vi "oldbis בדיקת מפל מתח בין הדקי הממסר תחת עומס 5.vi"(8 "error":errorcluster, 10 "lines":tag="PXI1Slot8/port0/line1", 11 "Path for Log":path) -> (0 "error IO":errorcluster, 1 "In Range?":bool, 2 "מפל מתח בין דקי הממסר תחת עומס":dbl, 3 "תוצאה זמנית":dbl)   [LabVIEW 2014]
uses:
  M9700 Driver/85/vi.lib/M9700 Modbus.llb/CTL Register Address.ctl
  M9700 Driver/86/vi.lib/M9700 Modbus.llb/CTL CMD Register.ctl
  <vilib>/Instr/_visa.llb/VISA Configure Serial Port (Instr).vi
  <vilib>/DAQmx/create/channels.llb/DAQmx Create Channel (DO-Digital Output).vi
  <vilib>/DAQmx/write.llb/DAQmx Write (Digital Bool 1Line 1Point).vi
panel:
  out "progress":dbl(slide) min=0.0 max=10.0 scale=0.0..10.0
  in  "stop":bool
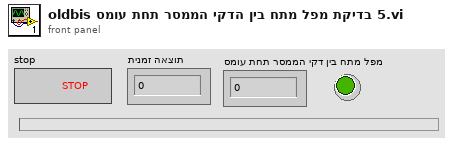
[diagram p1: front panel]
types:
  T1 = enum32{"Invalid", "Standard", "Closed", "Hidden", "Minimized", "Maximized"}
  T2 = typedef "CTL CMD Register.ctl" = u8
  T3 = typedef "CTL Register Address.ctl" = u16
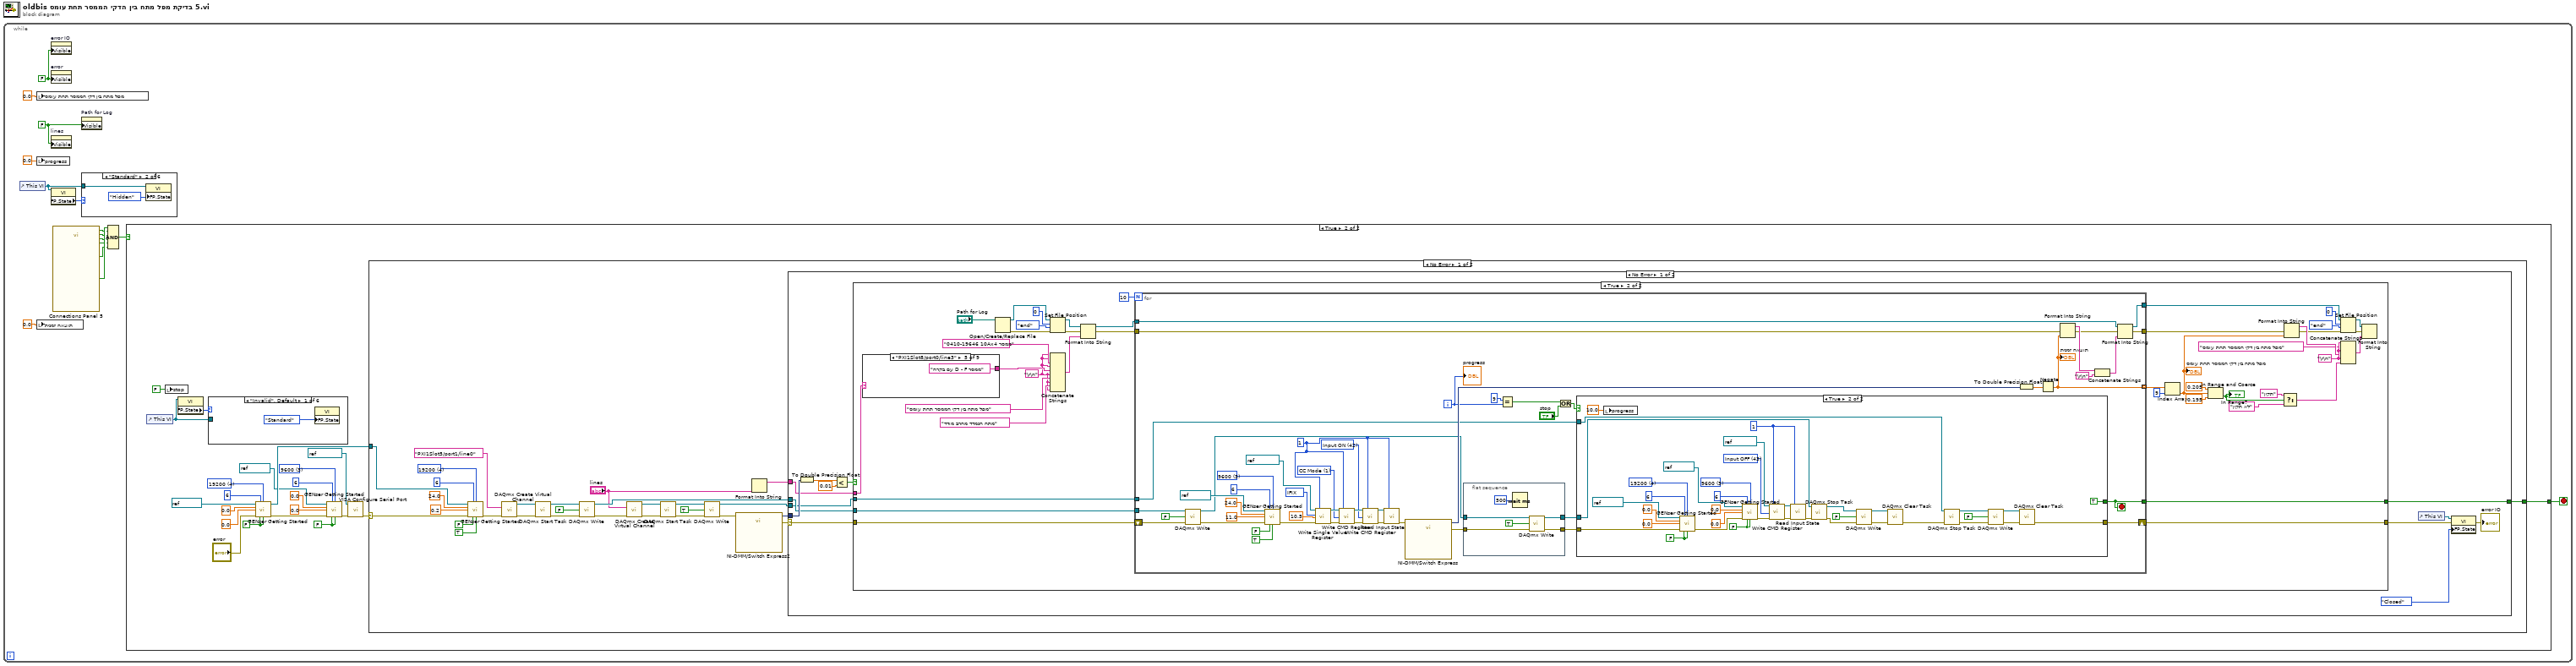
[diagram p0: block diagram]
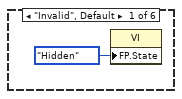
[diagram p2: hidden frame]
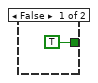
[diagram p7: hidden frame]
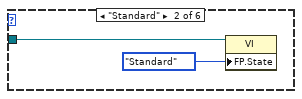
[diagram p8: hidden frame]
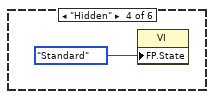
[diagram p10: hidden frame]
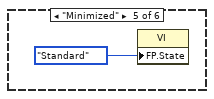
[diagram p11: hidden frame]
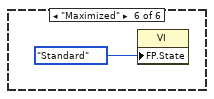
[diagram p12: hidden frame]
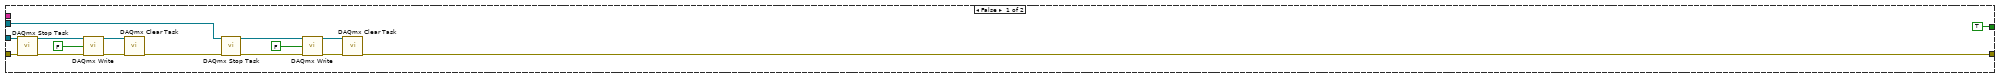
[diagram p13: hidden frame]
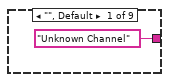
[diagram p14: hidden frame]
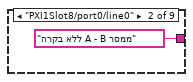
[diagram p15: hidden frame]
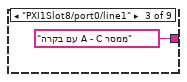
[diagram p16: hidden frame]
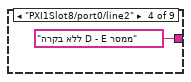
[diagram p17: hidden frame]
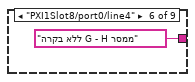
[diagram p18: hidden frame]
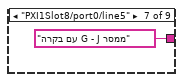
[diagram p19: hidden frame]
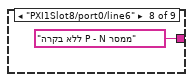
[diagram p20: hidden frame]
diagram:
  n1 = while {
    stop <- w15 stop-if-true
    w3 = FALSE ("Visible")
    w10 = FALSE ("Visible")
    n2 = control-ref of="This VI"() -> (w2:refnum<vi>)
    n3 = local write "מפל מתח בין דקי הממסר תחת עומס"(0.0 ("מפל מתח בין דקי הממסר תחת עומס")) -> ()
    n4 = local write "progress"(0.0 ("progress")) -> ()
    n5 = local write "תוצאה זמנית"(0.0 ("תוצאה זמנית")) -> ()
    n6 = property on="error IO" class="Clust (strict)"("Visible"=w10) -> ()  [unwired: 2 in, 2 out]
    n7 = property on="error" class="Clust (strict)"("Visible"=w10) -> ()  [unwired: 2 in, 2 out]
    n8 = property on="lines" class="DAQmxName"("Visible"=w3) -> ()  [unwired: 2 in, 2 out]
    n9 = property class="VI"(reference=w2) -> ("FP.State"=w1:T1)  [unwired: 1 in, 2 out]
    n10 = call "Connections Panel 5.vi"() -> ("Input Name 10"=w4:bool, "Input Name 6"=w8:bool, "Input Name 7"=w7:bool, "Input Name 8"=w6:bool, "Input Name 9"=w5:bool, "OK"=w9:bool)  [unwired: 13 in, 1 out]
    n11 = property on="Path for Log" class="Path"("Visible"=w3) -> ()  [unwired: 2 in, 2 out]
    n12 = case shown="\"Standard\"" w1 {
      tunnel: w2 -> [_ w17 _ _ _ _]
      frame "Invalid", Default {
        n13 = property class="VI"("FP.State"=T1."Hidden" ("Front Panel Window:State")) -> ()  [unwired: 2 in, 2 out]
      }
      frame "Standard" {
        n14 = property class="VI"(reference=w17, "FP.State"=T1."Hidden" ("Front Panel Window:State")) -> ()  [unwired: 1 in, 2 out]
      }
      frame "Closed" {
      }
      frame "Hidden" {
      }
      frame "Minimized" {
      }
      frame "Maximized" {
      }
    }
    n15 = Compound Arithmetic op=AND(w9, w8, w7, w6, w5, w4) -> (w14:bool)
    n16 = case shown="True" w14 {
      tunnel: [TRUE w28] -> w15
      frame False {
      }
      frame True {
        w24 = FALSE ("Reset (T)")
        w33 = u16 3 items=["1200", "2400", "4800", "9600", "19200"] ("BAUD")
        w23 = FALSE ("Output On (T)")
        w38 = u16 4 items=["1200", "2400", "4800", "9600", "19200"] ("BAUD")
        n17 = control-ref of="This VI"() -> (w20:refnum<vi>)
        n18 = local write "stop"(FALSE ("stop")) -> ()
        n19 = property class="VI"(reference=w20) -> ("FP.State"=w21:T1)  [unwired: 1 in, 2 out]
        n20 = case shown="\"Invalid\", Default" w21 {
          tunnel: w20 -> [_ w43 _ _ _ _]
          frame "Invalid", Default {
            n21 = property class="VI"("FP.State"=T1."Standard" ("Front Panel Window:State")) -> ()  [unwired: 2 in, 2 out]
          }
          frame "Standard" {
            n22 = property class="VI"(reference=w43, "FP.State"=T1."Standard" ("Front Panel Window:State")) -> ()  [unwired: 1 in, 2 out]
          }
          frame "Closed" {
          }
          frame "Hidden" {
            n23 = property class="VI"("FP.State"=T1."Standard" ("Front Panel Window:State")) -> ()  [unwired: 2 in, 2 out]
          }
          frame "Minimized" {
            n24 = property class="VI"("FP.State"=T1."Standard" ("Front Panel Window:State")) -> ()  [unwired: 2 in, 2 out]
          }
          frame "Maximized" {
            n25 = property class="VI"("FP.State"=T1."Standard" ("Front Panel Window:State")) -> ()  [unwired: 2 in, 2 out]
          }
        }
        n26 = call "GENser Getting Started.vi"("VISA"=refnum<visa-resource-name> "COM6", "GEN Addr"=i16 6, "BAUD"=w38, "Voltage Limit"=0.0, "Current Limit"=0.0, "error"="error", "Reset (T)"=w23, "Output On (T)"=w23) -> ("VISA out"=w40:refnum<visa-resource-name>, "error out"=w29:errorcluster)  [unwired: 4 in, 2 out]
        n27 = call "GENser Getting Started.vi"("VISA"=refnum<visa-resource-name> "COM4", "GEN Addr"=i16 6, "BAUD"=w33, "Voltage Limit"=0.0, "Current Limit"=0.0, "error"=w29, "Reset (T)"=w24, "Output On (T)"=w24) -> ("error out"=w26:errorcluster)  [unwired: 4 in, 3 out]
        n28 = call-poly "VISA Configure Serial Port"("VISA resource name"=refnum<visa-resource-name> "COM13", "error in (no error)"=w26) -> ("error out"=w25:errorcluster)  [unwired: 4 in, 9 out]
        n29 = case shown="No Error" w25 {
          selector: w25 -> [w73 _]
          tunnel: w40 -> [w76 _]
          tunnel: [w75 w255] -> w28
          frame No Error {
            w67 = u16 4 items=["1200", "2400", "4800", "9600", "19200"] ("BAUD")
            n30 = call "GENser Getting Started.vi"("VISA"=w76, "GEN Addr"=i16 6, "BAUD"=w67, "Voltage Limit"=24.0, "Current Limit"=0.2, "error"=w73, "Reset (T)"=FALSE, "Output On (T)"=TRUE) -> ("error out"=w61:errorcluster)  [unwired: 4 in, 3 out]
            n31 = call-poly <vilib>:"DAQmx Create Virtual Channel.vi"("lines"=tag "PXI1Slot5/port1/line0", "error in"=w61) -> ("task out"=w57:refnum<k21>, "error out"=w58:errorcluster)  [unwired: 12 in]
            n32 = call <vilib>:"DAQmx Start Task.vi"("task/channels in"=w57, "error in"=w58) -> ("task out"=w55:refnum<k21>, "error out"=w54:errorcluster)  [unwired: 12 in]
            n33 = call-poly <vilib>:"DAQmx Write.vi"("task/channels in"=w55, "data"=FALSE, "error in"=w54) -> ("task out"=w65:refnum<k21>, "error out"=w64:errorcluster)  [unwired: 10 in, 1 out]
            n34 = call-poly <vilib>:"DAQmx Create Virtual Channel.vi"("lines"="lines", "error in"=w64) -> ("task out"=w48:refnum<k21>, "error out"=w49:errorcluster)  [unwired: 12 in]
            n35 = call <vilib>:"DAQmx Start Task.vi"("task/channels in"=w48, "error in"=w49) -> ("task out"=w51:refnum<k21>, "error out"=w50:errorcluster)  [unwired: 12 in]
            n36 = call-poly <vilib>:"DAQmx Write.vi"("task/channels in"=w51, "data"=TRUE, "error in"=w50) -> ("task out"=w63:refnum<k21>, "error out"=w60:errorcluster)  [unwired: 10 in, 1 out]
            n37 = call "NI-DMM/Switch Express2"("error in"=w60) -> ("signals out"=w74:dynamicdata, "error out"=w59:errorcluster)  [unwired: 16 in, 1 out]
            n38 = Format Into String("lines") -> (resulting string=w66:string)  [unwired: 3 in, 1 out]
            n39 = case shown="No Error" w59 {
              selector: w59 -> [w87 _]
              tunnel: [w86 w250] -> w75
              tunnel: w74 -> [w89 _]
              tunnel: w65 -> [w80 _]
              tunnel: w66 -> [w78 _]
              tunnel: w63 -> [w77 _]
              frame No Error {
                n40 = To Double Precision Float(number=w89) -> (double precision float=w85:dbl)
                n41 = Less?(x=w85, y=0.01) -> (x < y?=w88:bool)
                n42 = case shown="True" w88 {
                  tunnel: w87 -> [w93 w108]
                  tunnel: [TRUE w146] -> w86
                  tunnel: [w90 w140] -> w81
                  tunnel: w80 -> [w92 w141]
                  tunnel: w78 -> [_ w110]
                  tunnel: w77 -> [w91 w109]
                  frame False {
                    n43 = call <vilib>:"DAQmx Stop Task.vi"("task/channels in"=w92, "error in"=w93) -> ("task out"=w104:refnum<k21>, "error out"=w102:errorcluster)  [unwired: 12 in]
                    n44 = call-poly <vilib>:"DAQmx Write.vi"("task/channels in"=w104, "data"=FALSE, "error in"=w102) -> ("task out"=w101:refnum<k21>, "error out"=w100:errorcluster)  [unwired: 10 in, 1 out]
                    n45 = call <vilib>:"DAQmx Clear Task.vi"("task in"=w101, "error in"=w100) -> ("error out"=w94:errorcluster)  [unwired: 13 in]
                    n46 = call <vilib>:"DAQmx Stop Task.vi"("task/channels in"=w91, "error in"=w94) -> ("task out"=w99:refnum<k21>, "error out"=w97:errorcluster)  [unwired: 12 in]
                    n47 = call-poly <vilib>:"DAQmx Write.vi"("task/channels in"=w99, "data"=FALSE, "error in"=w97) -> ("task out"=w96:refnum<k21>, "error out"=w95:errorcluster)  [unwired: 10 in, 1 out]
                    n48 = call <vilib>:"DAQmx Clear Task.vi"("task in"=w96, "error in"=w95) -> ("error out"=w90:errorcluster)  [unwired: 13 in]
                  }
                  frame True {
                    w127 = "\r\n"
                    w106 = "\r\n"
                    n49 = case shown="\"PXI1Slot8/port0/line3\"" w110 {
                      tunnel: ["Unknown Channel" "ללא בקרה A - B ממסר" "עם בקרה A - C ממסר" "ללא בקרה D - E ממסר" "עם בקרה D - F ממסר" "ללא בקרה G - H ממסר" "עם בקרה G - J ממסר" "ללא בקרה P - N ממסר" "עם בקרה P - L ממסר"] -> w107
                      frame "", Default {
                      }
                      frame "PXI1Slot8/port0/line0" {
                      }
                      frame "PXI1Slot8/port0/line1" {
                      }
                      frame "PXI1Slot8/port0/line2" {
                      }
                      frame "PXI1Slot8/port0/line3" {
                      }
                      frame "PXI1Slot8/port0/line4" {
                      }
                      frame "PXI1Slot8/port0/line5" {
                      }
                      frame "PXI1Slot8/port0/line6" {
                      }
                      frame "PXI1Slot8/port0/line7" {
                      }
                    }
                    n50 = Open/Create/Replace File(file path (use dialog)="Path for Log") -> (refnum out=w137:refnum<file>, error out=w136:errorcluster)  [unwired: 5 in, 1 out]
                    n51 = Set File Position(offset (in bytes) (0)=i64 0, refnum=w137, from (0:start)=enum16{"start", "end", "current"}."end", error in=w136) -> (refnum out=w133:refnum<file>, error out=w130:errorcluster)
                    n52 = Concatenate Strings(w106, w106, "0410-19646 10Ax4 ממסר", w106, w107, w106, "מפל מתח בין דקי הממסר תחת עומס", w106, "מתח הנמדד מהרב מודד", w106) -> (w135:string)
                    n53 = Format Into String(initial string=w133, error in=w130, w135) -> (resulting string=w128:refnum<file>, error out=w129:errorcluster)  [unwired: 1 in]
                    n54 = for {
                      N: 10 -> [_]
                      tunnel: [w180] -> w146
                      shift-right: [w177] -> w140
                      shift-left: w108 -> [w172]
                      tunnel: [w158] -> w145 mode=indexing
                      tunnel: w141 -> [w173]
                      tunnel: w129 -> [w162]
                      tunnel: w128 -> [w164]
                      tunnel: [w161] -> w121
                      tunnel: [w160] -> w112
                      tunnel: w109 -> [w159]
                      i -> [w176]
                      stop <- w180 stop-if-true
                      w188 = T2 42 items=["CC Mode"=1, "CV Mode"=2, "CW Mode"=3, "CR Mode"=4, "Short Mode"=26, "Set SysPara"=41, "Input ON"=42, "Input OFF"=43] ("CMD Register Value")
                      w191 = u8 1 ("Load Address")
                      w195 = T2 1 items=["CC Mode"=1, "CV Mode"=2, "CW Mode"=3, "CR Mode"=4, "Short Mode"=26, "Set SysPara"=41, "Input ON"=42, "Input OFF"=43] ("CMD Register Value")
                      w198 = T3 2561 items=["REMOTE"=1283, "ISTATE"=1296, "CMD"=2560, "IFIX"=2561, "UFIX"=2563, "PFIX"=2565, "RFIX"=2567, "IMAX"=2612, "UMAX"=2614, "PMAX"=2616, "U"=2816, "I"=2818, "MODEL"=2822, "EDITION"=2823] ("Register Address")
                      w203 = u16 3 items=["1200", "2400", "4800", "9600", "19200"] ("BAUD")
                      n55 = call-poly <vilib>:"DAQmx Write.vi"("task/channels in"=w173, "data"=FALSE, "error in"=w172) -> ("task out"=w171:refnum<k21>, "error out"=w170:errorcluster)  [unwired: 10 in, 1 out]
                      n56 = call "GENser Getting Started.vi"("VISA"=refnum<visa-resource-name> "COM4", "GEN Addr"=i16 6, "BAUD"=w203, "Voltage Limit"=24.0, "Current Limit"=11.0, "error"=w170, "Reset (T)"=FALSE, "Output On (T)"=TRUE) -> ("error out"=w193:errorcluster)  [unwired: 4 in, 3 out]
                      n57 = call "Write Single Value Register.vi"("VISA resource name"=refnum<visa-resource-name> "COM13", "Starting Address(HEX)"=w198, "Register Single Value"=sgl 10.5, "error in"=w193, "Load Address"=w191) -> ("VISA resource name out"=w197:refnum<visa-resource-name>, "error out"=w196:errorcluster)  [unwired: 13 out]
                      n58 = call "Write CMD Register.vi"("VISA resource name"=w197, "CMD Value"=w195, "error in"=w196, "Load Address"=w191) -> ("VISA resource name out"=w192:refnum<visa-resource-name>, "error out"=w189:errorcluster)  [unwired: 14 out]
                      n59 = call "Write CMD Register.vi"("VISA resource name"=w192, "CMD Value"=w188, "error in"=w189, "Load Address"=w191) -> ("VISA resource name out"=w190:refnum<visa-resource-name>, "error out"=w187:errorcluster)  [unwired: 14 out]
                      n60 = call "Read Input State.vi"("VISA resource name"=w190, "error in"=w187, "Load Address"=w191) -> ("error out"=w186:errorcluster)  [unwired: 16 out]
                      n61 = call "NI-DMM/Switch Express"("error in"=w186) -> ("signals out"=w185:dynamicdata, "error out"=w174:errorcluster)  [unwired: 16 in, 1 out]
                      n62 = flat-sequence {
                        tunnel: [w210] -> w175
                        tunnel: w174 -> [w209]
                        tunnel: w171 -> [w207]
                        tunnel: [w206] -> w168
                        frame #0 {
                          n63 = Wait (ms)(milliseconds to wait=u32 500) -> ()  [unwired: 1 out]
                          n64 = call-poly <vilib>:"DAQmx Write.vi"("task/channels in"=w207, "data"=TRUE, "error in"=w209) -> ("task out"=w206:refnum<k21>, "error out"=w210:errorcluster)  [unwired: 10 in, 1 out]
                        }
                      }
                      n65 = Equal?(x=9, y=w176) -> (x = y?=w182:bool)
                      n66 = Or(x=w182, y="stop") -> (x .or. y?=w183:bool)
                      n67 = case shown="True" w183 {
                        tunnel: [FALSE TRUE] -> w180
                        tunnel: w175 -> [w211 w238]
                        tunnel: [w211 w215] -> w177
                        tunnel: w168 -> [_ w221]
                        tunnel: w159 -> [_ w213]
                        frame False {
                        }
                        frame True {
                          w229 = u8 1 ("Load Address")
                          w232 = T2 43 items=["CC Mode"=1, "CV Mode"=2, "CW Mode"=3, "CR Mode"=4, "Short Mode"=26, "Set SysPara"=41, "Input ON"=42, "Input OFF"=43] ("CMD Register Value")
                          w236 = FALSE ("Reset (T)")
                          w242 = u16 3 items=["1200", "2400", "4800", "9600", "19200"] ("BAUD")
                          w235 = FALSE ("Reset (T)")
                          w245 = u16 4 items=["1200", "2400", "4800", "9600", "19200"] ("BAUD")
                          n68 = local write "progress"(10.0 ("progress")) -> ()
                          n69 = call "GENser Getting Started.vi"("VISA"=refnum<visa-resource-name> "COM6", "GEN Addr"=i16 6, "BAUD"=w245, "Voltage Limit"=0.0, "Current Limit"=0.0, "error"=w238, "Reset (T)"=w235, "Output On (T)"=w235) -> ("error out"=w237:errorcluster)  [unwired: 4 in, 3 out]
                          n70 = call "GENser Getting Started.vi"("VISA"=refnum<visa-resource-name> "COM4", "GEN Addr"=i16 6, "BAUD"=w242, "Voltage Limit"=0.0, "Current Limit"=0.0, "error"=w237, "Reset (T)"=w236, "Output On (T)"=w236) -> ("error out"=w234:errorcluster)  [unwired: 4 in, 3 out]
                          n71 = call "Write CMD Register.vi"("VISA resource name"=refnum<visa-resource-name> "COM13", "CMD Value"=w232, "error in"=w234, "Load Address"=w229) -> ("VISA resource name out"=w230:refnum<visa-resource-name>, "error out"=w233:errorcluster)  [unwired: 14 out]
                          n72 = call "Read Input State.vi"("VISA resource name"=w230, "error in"=w233, "Load Address"=w229) -> ("error out"=w222:errorcluster)  [unwired: 16 out]
                          n73 = call <vilib>:"DAQmx Stop Task.vi"("task/channels in"=w221, "error in"=w222) -> ("task out"=w227:refnum<k21>, "error out"=w225:errorcluster)  [unwired: 12 in]
                          n74 = call-poly <vilib>:"DAQmx Write.vi"("task/channels in"=w227, "data"=FALSE, "error in"=w225) -> ("task out"=w224:refnum<k21>, "error out"=w223:errorcluster)  [unwired: 10 in, 1 out]
                          n75 = call <vilib>:"DAQmx Clear Task.vi"("task in"=w224, "error in"=w223) -> ("error out"=w214:errorcluster)  [unwired: 13 in]
                          n76 = call <vilib>:"DAQmx Stop Task.vi"("task/channels in"=w213, "error in"=w214) -> ("task out"=w220:refnum<k21>, "error out"=w218:errorcluster)  [unwired: 12 in]
                          n77 = call-poly <vilib>:"DAQmx Write.vi"("task/channels in"=w220, "data"=FALSE, "error in"=w218) -> ("task out"=w217:refnum<k21>, "error out"=w216:errorcluster)  [unwired: 10 in, 1 out]
                          n78 = call <vilib>:"DAQmx Clear Task.vi"("task in"=w217, "error in"=w216) -> ("error out"=w215:errorcluster)  [unwired: 13 in]
                        }
                      }
                      n79 = To Double Precision Float(number=w185) -> (double precision float=w157:dbl)
                      n80 = Negate(x=w157) -> (-x=w158:dbl)
                      "תוצאה זמנית" <- w158
                      n81 = Format Into String(error in=w162, w158) -> (resulting string=w166:string, error out=w163:errorcluster)  [unwired: 2 in]
                      n82 = Concatenate Strings(w166, "\r\n") -> (w165:string)
                      n83 = Format Into String(initial string=w164, error in=w163, w165) -> (resulting string=w161:refnum<file>, error out=w160:errorcluster)  [unwired: 1 in]
                      "progress" <- w176
                    }
                    n84 = Index Array(array=w145, index=9) -> (element=w120:dbl)
                    "מפל מתח בין דקי הממסר תחת עומס" <- w120
                    n85 = In Range and Coerce(upper limit=0.205, x=w120, lower limit=0.195) -> (In Range?=w115:bool)  [unwired: 1 out]
                    "In Range?" <- w115
                    n86 = Select(t="תקין", s=w115, f="לא תקין") -> (s? t:f=w114:string)
                    n87 = Format Into String(error in=w112, w120) -> (resulting string=w119:string, error out=w113:errorcluster)  [unwired: 2 in]
                    n88 = Set File Position(offset (in bytes) (0)=i64 0, refnum=w121, from (0:start)=enum16{"start", "end", "current"}."end", error in=w113) -> (refnum out=w124:refnum<file>, error out=w123:errorcluster)
                    n89 = Concatenate Strings(w127, "מפל מתח בין דקי הממסר תחת עומס" ("string"), w127, w119, w127, w114) -> (w122:string)
                    n90 = Format Into String(initial string=w124, error in=w123, w122) -> ()  [unwired: 1 in, 2 out]
                  }
                }
                n91 = control-ref of="This VI"() -> (w83:refnum<vi>)
                n92 = property class="VI"(reference=w83, error in=w81, "FP.State"=T1."Closed" ("Front Panel Window:State")) -> (error out=→"error IO":errorcluster)  [unwired: 1 out]
              }
              frame Error {
                n93 = Two Button Dialog(message="בעיית דגימת נתונים ע\"י הכרטיס רב מודד", 1:"ביטול" ("F button name (\"Cancel\")"), 2:"נסה שוב" ("T button name (\"OK\")")) -> (T button?=w251:bool)
                n94 = Not(x=w251) -> (.not. x?=w250:bool)
              }
            }
          }
          frame Error {
            n95 = Two Button Dialog(message="בעיית תקשורת עם ספק קוח", 1:"ביטול" ("F button name (\"Cancel\")"), 2:"נסה שוב" ("T button name (\"OK\")")) -> (T button?=w256:bool)
            n96 = Not(x=w256) -> (.not. x?=w255:bool)
          }
        }
      }
    }
  }
